vi "Display Transmit Period.vi"(8 "error in":errorcluster, 10 "rate ref":refnum<vi>, 11 "label ref":T1 format="%.0x") -> (0 "error out":errorcluster, 3 "label ref out":T1 format="%.0x")   [LabVIEW 2024, in "AIM ARINC 429 System Explorer.lvlib" / "Implementation.lvlib"]
uses:
  Implementation.lvlib
  <vilib>/NI VeriStand/Custom Device API/Custom Device Item Ref.ctl
  Shared/Transfer Type.ctl
  <vilib>/NI VeriStand/Custom Device API/Custom Device API.lvlib
  Scripting/AIM/AIM ARINC 429 Scripting.lvlib
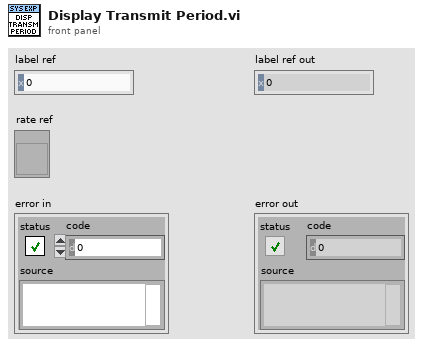
[diagram p1: front panel]
types:
  T1 = typedef "Custom Device API.lvlib/Custom Device Item Ref.ctl" = u64
  T2 = typedef "Direction.ctl" = enum16{"Rx", "Tx"}
  T3 = typedef "Transfer Type.ctl" = enum16{"Scheduled", "Acyclic", "Block", "Strobe"}
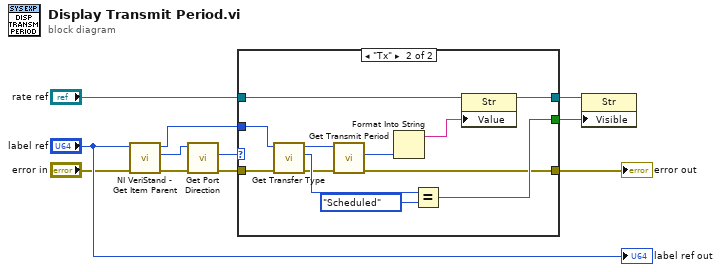
[diagram p0: block diagram]
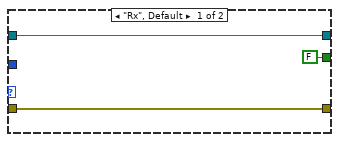
[diagram p2: hidden frame]
diagram:
  n1 = call <vilib>:"NI VeriStand - Get Item Parent.vi"("error in (no error)"="error in", "Item Ref in"="label ref") -> ("error out"=w8:errorcluster, "Parent Ref"=w10:T1, "Item Ref out"=w5:T1)  [unwired: 6 in, 1 out]
  n2 = call "Get Port Direction.vi"("error in"=w8, "port ref"=w10) -> ("error out"=w6:errorcluster, "direction"=w7:T2)  [unwired: 7 in, 1 out]
  n3 = case shown="\"Tx\"" w7 {
    tunnel: w6 -> [w12 w26]
    tunnel: w5 -> [_ w25]
    tunnel: "rate ref" -> [w14 w24]
    tunnel: [w14 w17] -> w3
    tunnel: [FALSE w16] -> w2
    tunnel: [w12 w15] -> w1
    frame "Rx", Default {
    }
    frame "Tx" {
      n4 = call "Get Transfer Type.vi"("error in"=w26, "label ref"=w25) -> ("error out"=w21:errorcluster, "transfer type"=w23:T3, "label ref out"=w20:T1)  [unwired: 7 in]
      n5 = call "Get Transmit Period.vi"("error in"=w21, "label ref"=w20) -> ("error out"=w15:errorcluster, "transmit period (us)"=w19:u32)  [unwired: 7 in, 1 out]
      n6 = Format Into String(w19) -> (resulting string=w18:string)  [unwired: 3 in, 1 out]
      n7 = Equal?(x=w23, y=Transfer_Type."Scheduled" ("x")) -> (x = y?=w16:bool)
      n8 = property class="Str"(reference=w24, "Value"=w18) -> (reference out=w17:refnum<vi>)  [unwired: 1 in, 1 out]
    }
  }
  "error out" <- w1
  n9 = property class="Str"(reference=w3, "Visible"=w2) -> ()  [unwired: 1 in, 2 out]
  "label ref out" <- "label ref"
